vi "PM100D_Write.vi"(2 "error in (no error)":errorcluster, 3 "Command":string, 4 "VISA in":refnum<visa-resource-name>="COM1") -> (0 "error out":errorcluster, 1 "VISA out":refnum<visa-resource-name>)   [LabVIEW 2014]
doc: "Writes a SCPI command to the connected instrument"
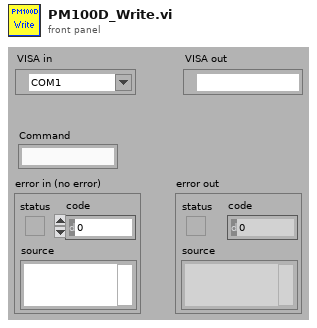
[diagram p1: front panel]
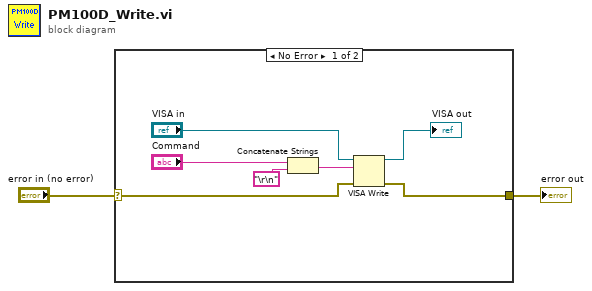
[diagram p0: block diagram]
diagram:
  n1 = case shown="No Error" "error in (no error)" {
    selector: "error in (no error)" -> [w3 w10]
    tunnel: [w6 w10] -> w2
    frame No Error {
      n2 = Concatenate Strings("Command", "\r\n") -> (w9:string)
      n3 = VISA Write(VISA resource name="VISA in", write buffer=w9, error in (no error)=w3) -> (VISA resource name out=→"VISA out":refnum<visa-resource-name>, error out=w6:errorcluster)  [unwired: 1 out]
    }
    frame Error {
    }
  }
  "error out" <- w2
